vi "Version 1_Read PID Settings.vi"(7 "Address (A)":string="A", 8 "error in":errorcluster, 11 "VISA Session In":refnum<visa-resource-name>="Alicat") -> (0 "error out":errorcluster, 1 "PID Loop Settings":T1={"P Gain"=0, "PID Type"=enum."PDF", "D Gain"=0, "I Gain"=0, "Valve Amount"=enum."Dual Valve"}, 3 "VISA Session Out":refnum<visa-resource-name>)   [LabVIEW 2020]
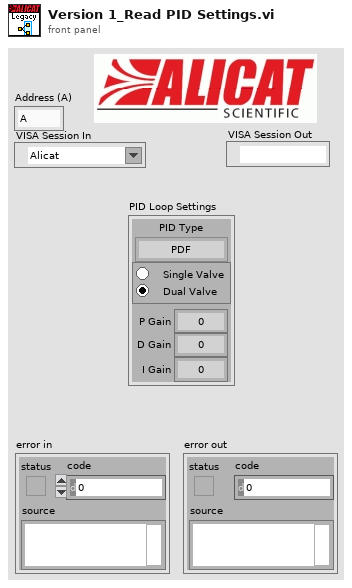
[diagram p1: front panel]
types:
  T1 = cluster{"P Gain":u16, "PID Type":enum8{"PDF", "PD2I"}, "D Gain":u16, "I Gain":u16, "Valve Amount":enum32{"Single Valve", "Dual Valve"}}
  T2 = cluster{"Valve Amount":enum8{"Single Valve", "Dual Valve"}, "PID Type":enum8{"PDF", "PD2I"}, "Valve Offset":i32, "P Gain":i32, "D Gain":i32, "I Gain":i32}
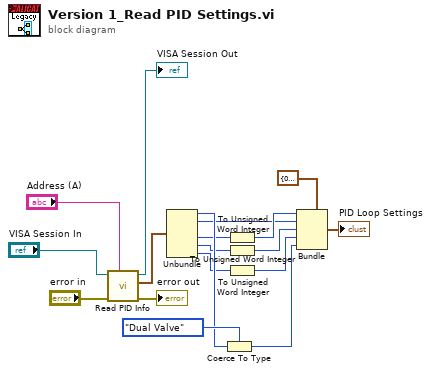
[diagram p0: block diagram]
diagram:
  n1 = call "Read PID Info.vi"("VISA Session In"="VISA Session In", "error in"="error in", "Unit ID (A)"="Address (A)") -> ("VISA Session Out"=→"VISA Session Out":refnum<visa-resource-name>, "PID Settings"=w11:T2, "error out"=→"error out":errorcluster)  [unwired: 5 in]
  n2 = Unbundle(w11) -> ("Valve Amount"=w8:enum8{"Single Valve", "Dual Valve"}, "PID Type"=w1:enum8{"PDF", "PD2I"}, "P Gain"=w7:i32, "D Gain"=w6:i32, "I Gain"=w5:i32)  [unwired: 1 out]
  n3 = Coerce To Type(0:w8, 1:enum32{"Single Valve", "Dual Valve"}."Dual Valve" ("Valve Amount")) -> (2:w10:enum32{"Single Valve", "Dual Valve"})
  n4 = To Unsigned Word Integer(number=w7) -> (unsigned 16bit integer=w3:u16)
  n5 = To Unsigned Word Integer(number=w6) -> (unsigned 16bit integer=w2:u16)
  n6 = To Unsigned Word Integer(number=w5) -> (unsigned 16bit integer=w4:u16)
  n7 = Bundle(cluster=T1 {"P Gain"=0, "PID Type"=enum."PDF", "D Gain"=0, "I Gain"=0, "Valve Amount"=enum."Dual Valve"} ("PID Loop Settings"), "P Gain"=w3, "PID Type"=w1, "D Gain"=w2, "I Gain"=w4, "Valve Amount"=w10) -> (→"PID Loop Settings":T1)
